vi "Update_2layer_Wx.vi"(0 "Target_OutX":dbl, 1 "2layer_OutX 2":dbl, 2 "Learning rate":dbl, 3 "Array_Out_hx":dbl[](array[numeric]), 4 "Weights_2layer":dbl[](array[numeric])) -> (5 "Weights_2layer_updated":dbl[](array[numeric]))   [LabVIEW 2016]
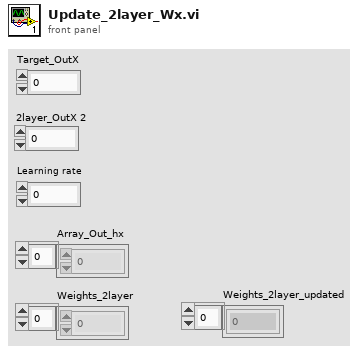
[diagram p1: front panel]
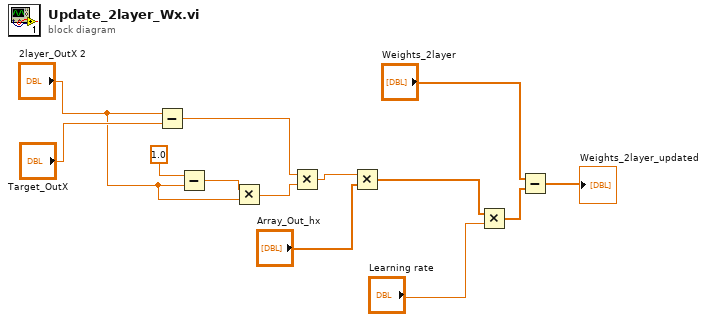
[diagram p0: block diagram]
diagram:
  n1 = Subtract(x="2layer_OutX 2", y="Target_OutX") -> (x-y=w10:dbl)
  n2 = Subtract(x=1.0, y="2layer_OutX 2") -> (x-y=w12:dbl)
  n3 = Multiply(x=w12, y="2layer_OutX 2") -> (x*y=w9:dbl)
  n4 = Multiply(x=w10, y=w9) -> (x*y=w5:dbl)
  n5 = Multiply(x=w5, y="Array_Out_hx") -> (x*y=w3:dbl[])
  n6 = Multiply(x=w3, y="Learning rate") -> (x*y=w8:dbl[])
  n7 = Subtract(x="Weights_2layer", y=w8) -> (x-y=→"Weights_2layer_updated":dbl[])
